vi "Get Data.vi"(8 "error in (no error)":errorcluster, 10 "Bus In":refnum<class "Bus.lvclass">, 11 "Single Query in":refnum<class "Single Query.lvclass">) -> (0 "error out":errorcluster, 1 "String Read":string, 2 "Bus Out":refnum<class "Bus.lvclass">, 3 "Single Query out":refnum<class "Single Query.lvclass">)   [LabVIEW 2024, in "Single Query.lvclass"]
doc: "Single Query.lvclass:Get Data.vi\n\nThis VI does a Query and a Response for the Single Query instance of the Query class.\n\nInstrument Communication Module Version 1.0\nDecember, 2017 Original Code Consulting David Thomson\n www.originalcode.com"
uses:
  Single Query.lvclass
  Bus/Bus.lvclass
  Single Query.lvclass/Single Query.ctl
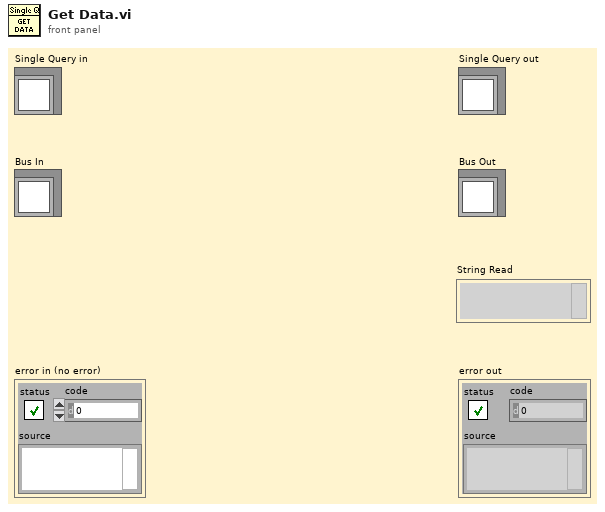
[diagram p1: front panel]
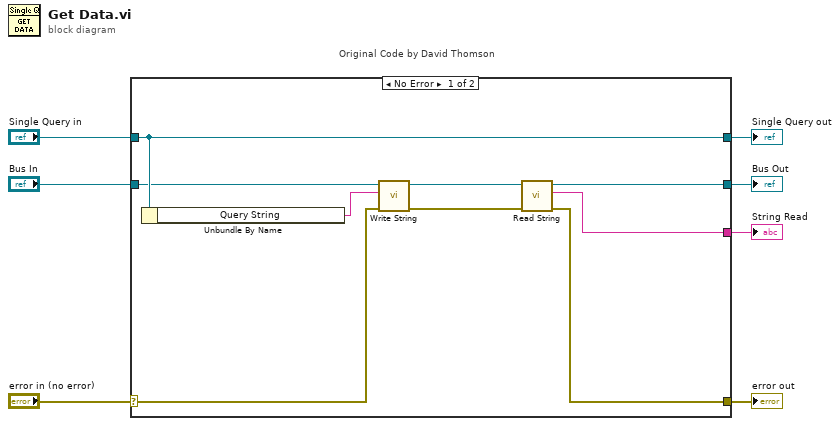
[diagram p0: block diagram]
diagram:
  n1 = case "Original Code by David Thomson" shown="No Error" "error in (no error)" {
    selector: "error in (no error)" -> [w9 w19]
    tunnel: [w15 w19] -> w6
    tunnel: [w13 w18] -> w4
    tunnel: "Single Query in" -> [w13 w18]
    tunnel: [w16 w17] -> w3
    tunnel: "Bus In" -> [w12 w17]
    tunnel: [w14 _] -> w1
    frame No Error {
      n2 = Unbundle By Name(w13) -> ("Query String"=w10:string)
      n3 = call-dynamic "Write String.vi"("error in (no error)"=w9, "String"=w10, "Bus in"=w12) -> ("error out"=w8:errorcluster, "Bus out"=w11:refnum<class "Bus.lvclass">)  [unwired: 7 in]
      n4 = call-dynamic "Read String.vi"("error in (no error)"=w8, "Bus in"=w11) -> ("error out"=w15:errorcluster, "String Read"=w14:string, "Bus out"=w16:refnum<class "Bus.lvclass">)  [unwired: 6 in, 1 out]
    }
    frame Error {
    }
  }
  "error out" <- w6
  "Single Query out" <- w4
  "Bus Out" <- w3
  "String Read" <- w1
